vi "LogData.vi"(0 "LotData in":refnum<class "LotData.lvclass">, 1 "20mA Spectra":cluster{"Wavelength":dbl[], "EL Spectrum":dbl[]}, 2 "50mA Spectra":cluster{"Wavelength":dbl[], "EL Spectrum":dbl[]}, 3 "error in (no error)":errorcluster, 4 "Data In":T1 {"50mA Data"."Current,mA" format="%_6g"; "50mA Data"."WL" format="%_6g"; "50mA Data"."Voltage" format="%_6g"; "50mA Data"."Power" format="%_6g"; "20mA Data"."Reverse" format="%#_3g"; "20mA Data"."Current,mA" format="%_6g"; "20mA Data"."Knee Current" format="%#_3g"; "20mA Data"."WL" format="%_6g"; "20mA Data"."Voltage" format="%_6g"; "20mA Data"."Power" format="%_5g"}) -> (7 "LotData out":refnum<class "LotData.lvclass">, 8 "LogData":string, 9 "Error":bool, 10 "error out":errorcluster)   [LabVIEW 2012, in "LotData.lvclass"]
uses:
  LotData.lvclass
  Controls/TestData.ctl
panel:
  out "LogData_50":string
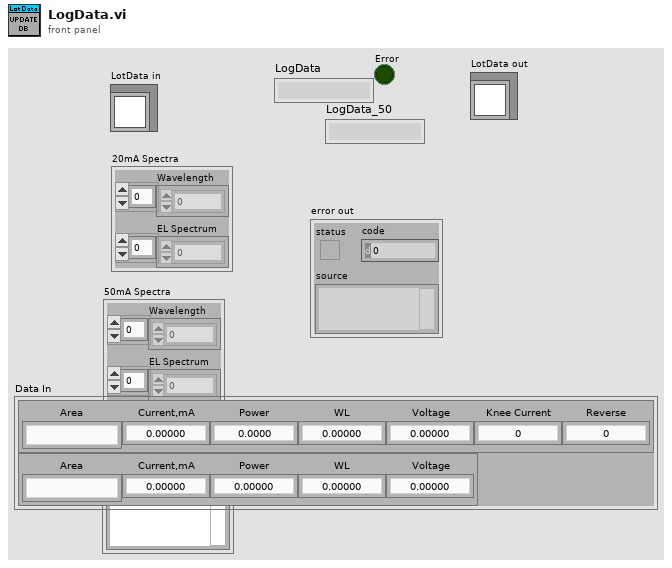
[diagram p1: front panel]
types:
  T1 = typedef "TestData.ctl" = cluster{"20mA Data":cluster{"Area":string, "Current,mA":dbl, "Power":dbl, "WL":dbl, "Voltage":dbl, "Knee Current":dbl, "Reverse":dbl}, "50mA Data":cluster{"Area":string, "Current,mA":dbl, "Power":dbl, "WL":dbl, "Voltage":dbl}}
  T2 = cluster{"Area":string, "Current,mA":dbl, "Power":dbl, "WL":dbl, "Voltage":dbl}
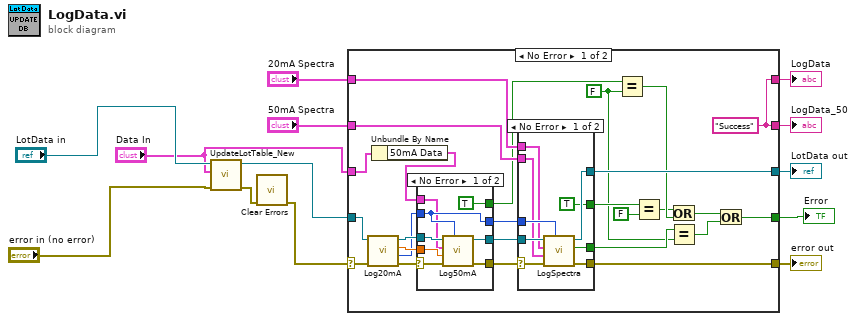
[diagram p0: block diagram]
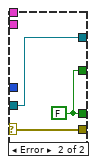
[diagram p2: hidden frame]
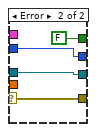
[diagram p3: hidden frame]
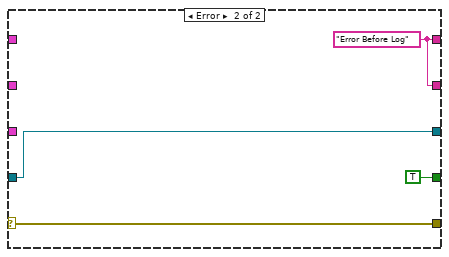
[diagram p4: hidden frame]
diagram:
  n1 = call-dynamic "UpdateLotTable_New.vi"("error in (no error)"="error in (no error)", "input cluster"="Data In", "LotData in"="LotData in") -> ("error out"=w4:errorcluster, "LotData out"=w2:refnum<class "LotData.lvclass">)  [unwired: 7 in]
  n2 = call <vilib>:"Clear Errors.vi"("error in (no error)"=w4) -> ("error out"=w3:errorcluster)  [unwired: 6 in]
  n3 = case shown="No Error" w3 {
    selector: w3 -> [w38 w67]
    tunnel: [w27 w67] -> w13
    tunnel: [w28 w66] -> w12
    tunnel: w2 -> [w39 w66]
    tunnel: [w21 w65] -> w11
    tunnel: "50mA Spectra" -> [w29 _]
    tunnel: "20mA Spectra" -> [w30 _]
    tunnel: "Data In" -> [w15 _]
    tunnel: [w21 w65] -> w8
    tunnel: [w16 TRUE] -> w7
    frame No Error {
      w21 = "Success" ("LogData")
      w19 = FALSE ("y")
      n4 = call-dynamic "Log20mA.vi"("error in (no error)"=w38, "LotData in"=w39) -> ("error out"=w37:errorcluster, "area"=w34:i32, "reverse"=w35:dbl, "LotData out"=w36:refnum<class "LotData.lvclass">)  [unwired: 6 in]
      n5 = Unbundle By Name(w15) -> ("50mA Data"=w14:T2)
      n6 = case shown="No Error" w37 {
        selector: w37 -> [w58 w63]
        tunnel: w36 -> [w59 w62]
        tunnel: w35 -> [w57 _]
        tunnel: w34 -> [w54 w61]
        tunnel: [w56 w63] -> w31
        tunnel: [w55 w62] -> w33
        tunnel: [w54 w61] -> w32
        tunnel: [TRUE FALSE] -> w24
        tunnel: w14 -> [w52 _]
        frame No Error {
          n7 = call-dynamic "Log50mA.vi"("Area"=w54, "error in (no error)"=w58, "Reverse"=w57, "50mA Data"=w52, "LotData in"=w59) -> ("error out"=w56:errorcluster, "LotData out"=w55:refnum<class "LotData.lvclass">)  [unwired: 5 in]
        }
        frame Error {
        }
      }
      n8 = case shown="No Error" w31 {
        selector: w31 -> [w44 w51]
        tunnel: w33 -> [w48 w50]
        tunnel: w32 -> [w47 _]
        tunnel: w30 -> [w46 _]
        tunnel: w29 -> [w45 _]
        tunnel: [w43 w51] -> w27
        tunnel: [w42 w50] -> w28
        tunnel: [TRUE w49] -> w26
        tunnel: [w40 w49] -> w20
        frame No Error {
          n9 = call-dynamic "LogSpectra.vi"("Area"=w47, "error in (no error)"=w44, "50mA Spectra"=w45, "20mA Spectra"=w46, "LotData in"=w48) -> ("error out"=w43:errorcluster, "Boolean"=w40:bool, "LotData out"=w42:refnum<class "LotData.lvclass">)  [unwired: 4 in]
        }
        frame Error {
          w49 = FALSE
        }
      }
      n10 = Equal?(x=w24, y=w19) -> (x = y?=w23:bool)
      n11 = Equal?(x=w26, y=FALSE) -> (x = y?=w22:bool)
      n12 = Or(x=w22, y=w23) -> (x .or. y?=w18:bool)
      n13 = Equal?(x=w20, y=w19) -> (x = y?=w17:bool)
      n14 = Or(x=w18, y=w17) -> (x .or. y?=w16:bool)
    }
    frame Error {
      w65 = "Error Before Log" ("LogData")
    }
  }
  "error out" <- w13
  "LotData out" <- w12
  "LogData" <- w11
  "LogData_50" <- w8
  "Error" <- w7
